vi "Get Parent Interface.vi"(8 "error in (no error)":errorcluster, 10 "Test Class Path":path) -> (0 "error out":errorcluster, 2 "Path":path)   [LabVIEW 2020, in "Responsive Mock Class Generator Test.lvclass"]
uses:
  Responsive Mock Class Generator Test.lvclass
  Responsive Mock Class Generator Test.lvclass/Responsive Mock Class Generator Test.ctl
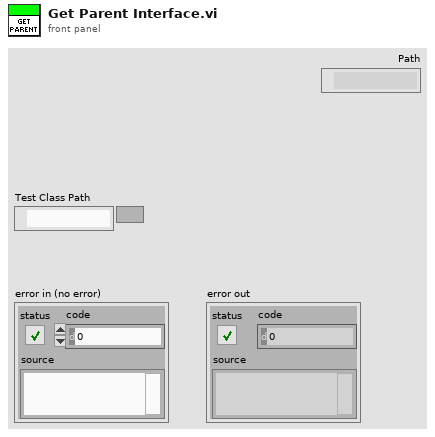
[diagram p1: front panel]
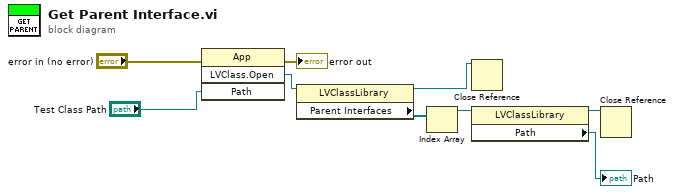
[diagram p0: block diagram]
diagram:
  n1 = invoke class="App" method="LVClass.Open"(error in="error in (no error)", "Path"="Test Class Path") -> (error out=→"error out":errorcluster, "LVClass.Open"=w6:refnum<vi>)  [unwired: 2 in, 2 out]
  n2 = property class="LVClassLibrary"(reference=w6) -> (reference out=w3:refnum<vi>, "Parent Interfaces"=w5:refnum<vi>[])  [unwired: 1 in, 1 out]
  n3 = Index Array(array=w5) -> (element=w1:refnum<vi>)  [unwired: 1 in]
  n4 = Close Reference(reference=w3) -> ()  [unwired: 1 in, 1 out]
  n5 = property class="LVClassLibrary"(reference=w1) -> (reference out=w2:refnum<vi>, "Path"=→"Path":path)  [unwired: 1 in, 1 out]
  n6 = Close Reference(reference=w2) -> ()  [unwired: 1 in, 1 out]
